vi "Phase atan2.vi"(11 "Feedback In":T1) -> (3 "atan2(y,x)":dbl)   [LabVIEW 2018]
uses:
  Phase Calculator Feedback Cluster.ctl
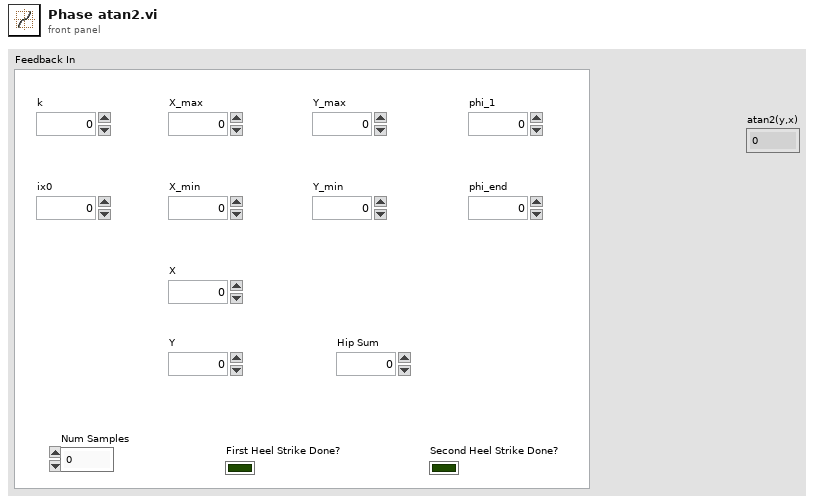
[diagram p1: front panel]
types:
  T1 = typedef "Phase Calculator Feedback Cluster.ctl" = cluster{"k":dbl, "ix0":dbl, "X_max":dbl, "X_min":dbl, "Y_max":dbl, "Y_min":dbl, "Y":dbl, "Hip Sum":dbl, "Num Samples":dbl, "First Heel Strike Done?":bool, "Second Heel Strike Done?":bool, "phi_1":dbl, "phi_end":dbl, "X":dbl}
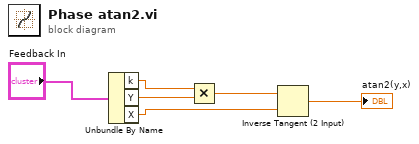
[diagram p0: block diagram]
diagram:
  n1 = Unbundle By Name("Feedback In") -> ("k"=w5:dbl, "Y"=w4:dbl, "X"=w2:dbl)
  n2 = Multiply(x=w5, y=w4) -> (x*y=w3:dbl)
  n3 = Inverse Tangent (2 Input)(1:w2, 2:w3) -> (0:→"atan2(y,x)":dbl)
